vi "main_layout.vi"(7 "layout_mode":T1, 8 "error in":errorcluster) -> (0 "error out":errorcluster)   [LabVIEW 2016]
uses:
  main_display_modes.ctl
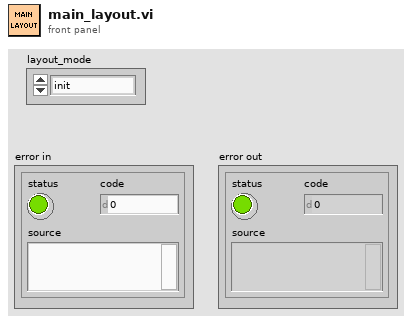
[diagram p1: front panel]
types:
  T1 = typedef "main_display_modes.ctl" = enum16{"init", "after_config", "after_start", "end"}
  T2 = enum8{"Enabled", "Disabled", "Disabled and Grayed Out"}
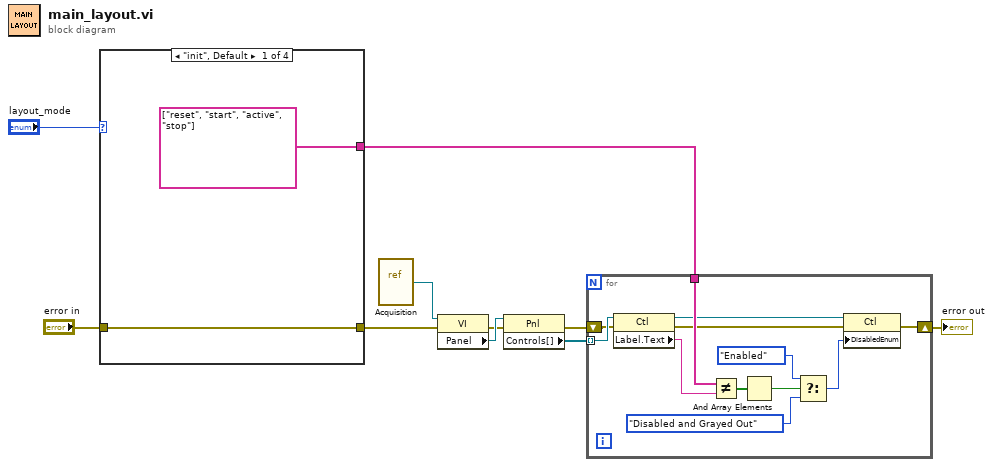
[diagram p0: block diagram]
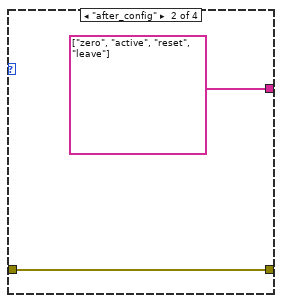
[diagram p2: hidden frame]
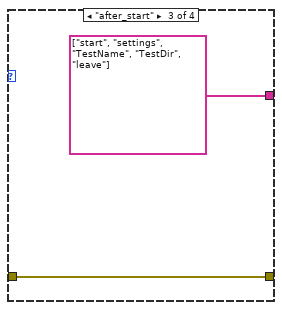
[diagram p3: hidden frame]
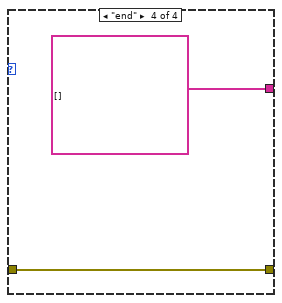
[diagram p4: hidden frame]
diagram:
  n1 = case shown="\"init\", Default" "layout_mode" {
    tunnel: [string[] ["reset", "start", "active", "stop"] string[] ["zero", "active", "reset", "leave"] string[] ["start", "settings", "TestName", "TestDir", "leave"] string[] []] -> w4
    tunnel: [w11 w13 w15 w17] -> w2
    tunnel: "error in" -> [w11 w13 w15 w17]
    frame "init", Default {
    }
    frame "after_config" {
    }
    frame "after_start" {
    }
    frame "end" {
    }
  }
  n2 = vi-ref "Acquisition.vi"() -> (w7:refnum<vi>)
  n3 = property class="VI"(reference=w7, error in=w2) -> (error out=w8:errorcluster, "Panel"=w9:refnum<vi>)  [unwired: 1 out]
  n4 = property class="Pnl"(reference=w9, error in=w8) -> (error out=w5:errorcluster, "Controls[]"=w6:refnum<vi>[])  [unwired: 1 out]
  n5 = for {
    tunnel: w6 -> [w30] mode=indexing
    shift-right: [w19] -> w3
    shift-left: w5 -> [w29]
    tunnel: w4 -> [w27]
    n6 = property class="Ctl"(reference=w30, error in=w29) -> (reference out=w24:refnum<vi>, error out=w25:errorcluster, "Label.Text"=w28:string)
    n7 = Not Equal?(x=w27, y=w28) -> (x != y?=w26:bool[])
    n8 = And Array Elements(Boolean array=w26) -> (logical AND=w23:bool)
    n9 = Select(t=T2."Enabled" ("Disabled"), s=w23, f=T2."Disabled and Grayed Out" ("Disabled")) -> (s? t:f=w20:T2)
    n10 = property class="Ctl"(reference=w24, error in=w25, "DisabledEnum"=w20) -> (error out=w19:errorcluster)  [unwired: 1 out]
  }
  "error out" <- w3
